vi "PeakLocations.vi"(8 "Threshold":dbl, 9 "width":i32=3 min=3, 10 "peaks/valleys":enum32{"Peaks", "Valleys"}(ring), 11 "Data Array":dbl[][](array[numeric])) -> (3 "Locations":dbl[][](array[numeric]))   [LabVIEW 2014]
uses:
  <vilib>/Analysis/NI_AAL_SigProc.lvlib
panel:
  # "Inputs"
  # "Outputs"
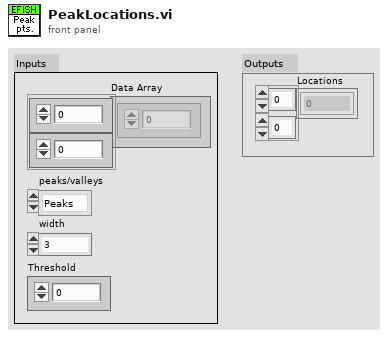
[diagram p1: front panel]
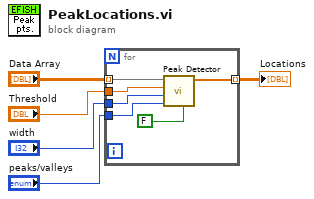
[diagram p0: block diagram]
diagram:
  n1 = for {
    tunnel: "Data Array" -> [w11] mode=indexing
    tunnel: "Threshold" -> [w10]
    tunnel: "peaks/valleys" -> [w9]
    tunnel: "width" -> [w7]
    tunnel: [w6] -> w1 mode=indexing
    n2 = call <vilib>:"Peak Detector.vi"("end of data (T)"=FALSE, "peaks/valleys"=w9, "width"=w7, "threshold"=w10, "X"=w11) -> ("Locations"=w6:dbl[])  [unwired: 2 in, 4 out]
  }
  "Locations" <- w1
